vi "provide_note_book_info.vi"(8 "error in (no error)":errorcluster, 10 "notebook string in":string, 11 "ScanModeDL090923Scaffold in":refnum<class "ImagingModeMG091111IntrinsicImaging.lvclass">) -> (0 "error out":errorcluster, 2 "notebook string out":string, 3 "ScanModeDL090923Scaffold out":refnum<class "ImagingModeMG091111IntrinsicImaging.lvclass">)   [LabVIEW 2010, in "ImagingModeMG091111IntrinsicImaging.lvclass"]
uses:
  ImagingModeMG091111IntrinsicImaging.lvclass
  ImagingModeDL091001Scaffold/ImagingModeDL091001Scaffold/ImagingModeDL091001Scaffold.lvclass
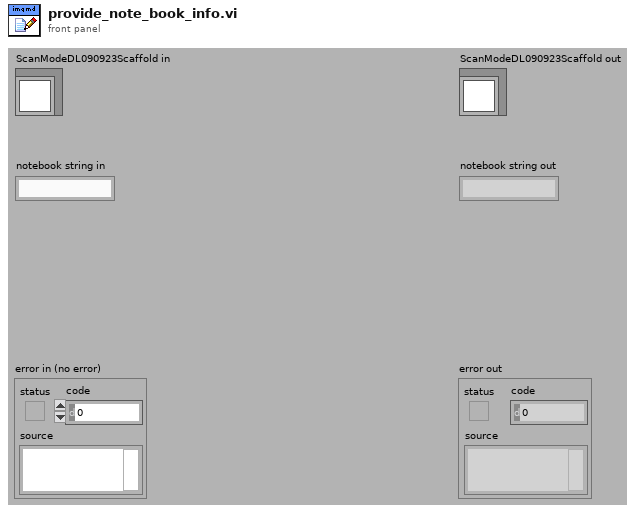
[diagram p1: front panel]
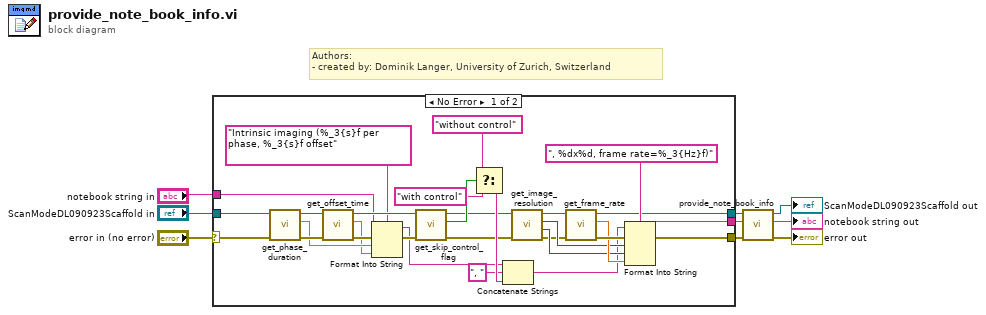
[diagram p0: block diagram]
diagram:
  # "Authors: \n- created by: Dominik Langer, University of Zurich, Switzerland"
  n1 = case shown="No Error" "error in (no error)" {
    selector: "error in (no error)" -> [w39 w42]
    tunnel: "notebook string in" -> [w24 w40]
    tunnel: "ScanModeDL090923Scaffold in" -> [w38 w41]
    tunnel: [w14 w42] -> w3
    tunnel: [w13 w41] -> w2
    tunnel: [w11 w40] -> w1
    frame No Error {
      n2 = call-dynamic "get_phase_duration.vi"("error in (no error)"=w39, "ScanModeMG091111IntrinsicImaging in"=w38) -> ("error out"=w23:errorcluster, "phase duration"=w21:dbl[unit], "ScanModeMG091111IntrinsicImaging out"=w37:refnum<class "ImagingModeMG091111IntrinsicImaging.lvclass">)  [unwired: 7 in]
      n3 = call-dynamic "get_offset_time.vi"("error in (no error)"=w23, "ScanModeMG091111IntrinsicImaging in"=w37) -> ("error out"=w22:errorcluster, "offset time"=w20:dbl[unit], "ScanModeMG091111IntrinsicImaging out"=w35:refnum<class "ImagingModeMG091111IntrinsicImaging.lvclass">)  [unwired: 7 in]
      n4 = Format Into String(format string="Intrinsic imaging (%_3{s}f per  phase, %_3{s}f offset", initial string=w24, error in=w22, w21, w20) -> (resulting string=w30:string, error out=w36:errorcluster)
      n5 = call-dynamic "get_skip_control_flag.vi"("error in (no error)"=w36, "ScanModeMG091111IntrinsicImaging in"=w35) -> ("error out"=w29:errorcluster, "skip control?"=w34:bool, "ScanModeMG091111IntrinsicImaging out"=w28:refnum<class "ImagingModeMG091111IntrinsicImaging.lvclass">)  [unwired: 7 in]
      n6 = Select(t="without control" ("string"), s=w34, f="with control" ("string")) -> (s? t:f=w31:string)
      n7 = Concatenate Strings(w30, ", " ("string"), w31) -> (w12:string)
      n8 = call-dynamic "get_image_resolution.vi"("error in (no error)"=w29, "ScanModeMG091111IntrinsicImaging in"=w28) -> ("error out"=w15:errorcluster, "ImageHeight"=w16:i32, "ImageWidth"=w17:i32, "ScanModeMG091111IntrinsicImaging out"=w27:refnum<class "ImagingModeMG091111IntrinsicImaging.lvclass">)  [unwired: 6 in]
      n9 = call-dynamic "get_frame_rate.vi"("error in (no error)"=w15, "ScanModeMG091111IntrinsicImaging in"=w27) -> ("error out"=w26:errorcluster, "frame rate"=w18:dbl[unit], "ScanModeMG091111IntrinsicImaging out"=w13:refnum<class "ImagingModeMG091111IntrinsicImaging.lvclass">)  [unwired: 7 in]
      n10 = Format Into String(format string=", %dx%d, frame rate=%_3{Hz}f)", initial string=w12, error in=w26, w17, w16, w18) -> (resulting string=w11:string, error out=w14:errorcluster)
    }
    frame Error {
    }
  }
  n11 = call-parent "provide_note_book_info.vi"("error in (no error)"=w3, "notebook string in"=w1, "GenericPlugin in"=w2) -> ("error out"=→"error out":errorcluster, "notebook string out"=→"notebook string out":string, "GenericPlugin out"=→"ScanModeDL090923Scaffold out":refnum<class "ImagingModeMG091111IntrinsicImaging.lvclass">)  [unwired: 6 in]
